vi "DisplayExternals.vi"(7 "AcroPDF":refnum<k7>(container), 8 "error in (no error)":errorcluster, 10 "Dynamic data":T1, 11 "Input parameters":T2={"Measurement type"=enum."Test", "Sensor type"=enum."HPK_8in_256", "Identifier"="test.txt", "Open after execution?"=FALSE, "Plot after execution?"=FALSE, "Display channel"=0, "Voltage Delay (s)"=0.5, "Switch Delay (s)"=0.01, "VISA resource name source"="", "VISA resource name DMM"="", "VISA resource name LCR"="", "Compliance  Level (uA)"=10.0, "Voltage Limit (V)"=1000.0, "Data storage location"="", "Scan voltages"="", "Use source as DMM?"=FALSE, "Single channel?"=FALSE, "LCR signal frequenzy (Hz)"=10.0, "DMM device"=enum."Keithley2001", "Sampling number"=1, "Use env. sensors on"=enum."Sensirion sht1x/7x"} {"Voltage Limit (V)" format="%#_13g"; "Voltage Delay (s)" format="%#_13g"; "Switch Delay (s)" format="%#_13g"}) -> (0 "error out":errorcluster, 2 "Dynamic data":T1, 3 "Input parameters":T2={"Measurement type"=enum."Test", "Sensor type"=enum."HPK_8in_256", "Identifier"="test.txt", "Open after execution?"=FALSE, "Plot after execution?"=FALSE, "Display channel"=0, "Voltage Delay (s)"=0.5, "Switch Delay (s)"=0.01, "VISA resource name source"="", "VISA resource name DMM"="", "VISA resource name LCR"="", "Compliance  Level (uA)"=10.0, "Voltage Limit (V)"=1000.0, "Data storage location"="", "Scan voltages"="", "Use source as DMM?"=FALSE, "Single channel?"=FALSE, "LCR signal frequenzy (Hz)"=10.0, "DMM device"=enum."Keithley2001", "Sampling number"=1, "Use env. sensors on"=enum."Sensirion sht1x/7x"} {"Voltage Limit (V)" format="%#_13g"; "Voltage Delay (s)" format="%#_13g"; "Switch Delay (s)" format="%#_13g"})   [LabVIEW 2016]
uses:
  Input_parameters.ctl
  Dynamic_data.ctl
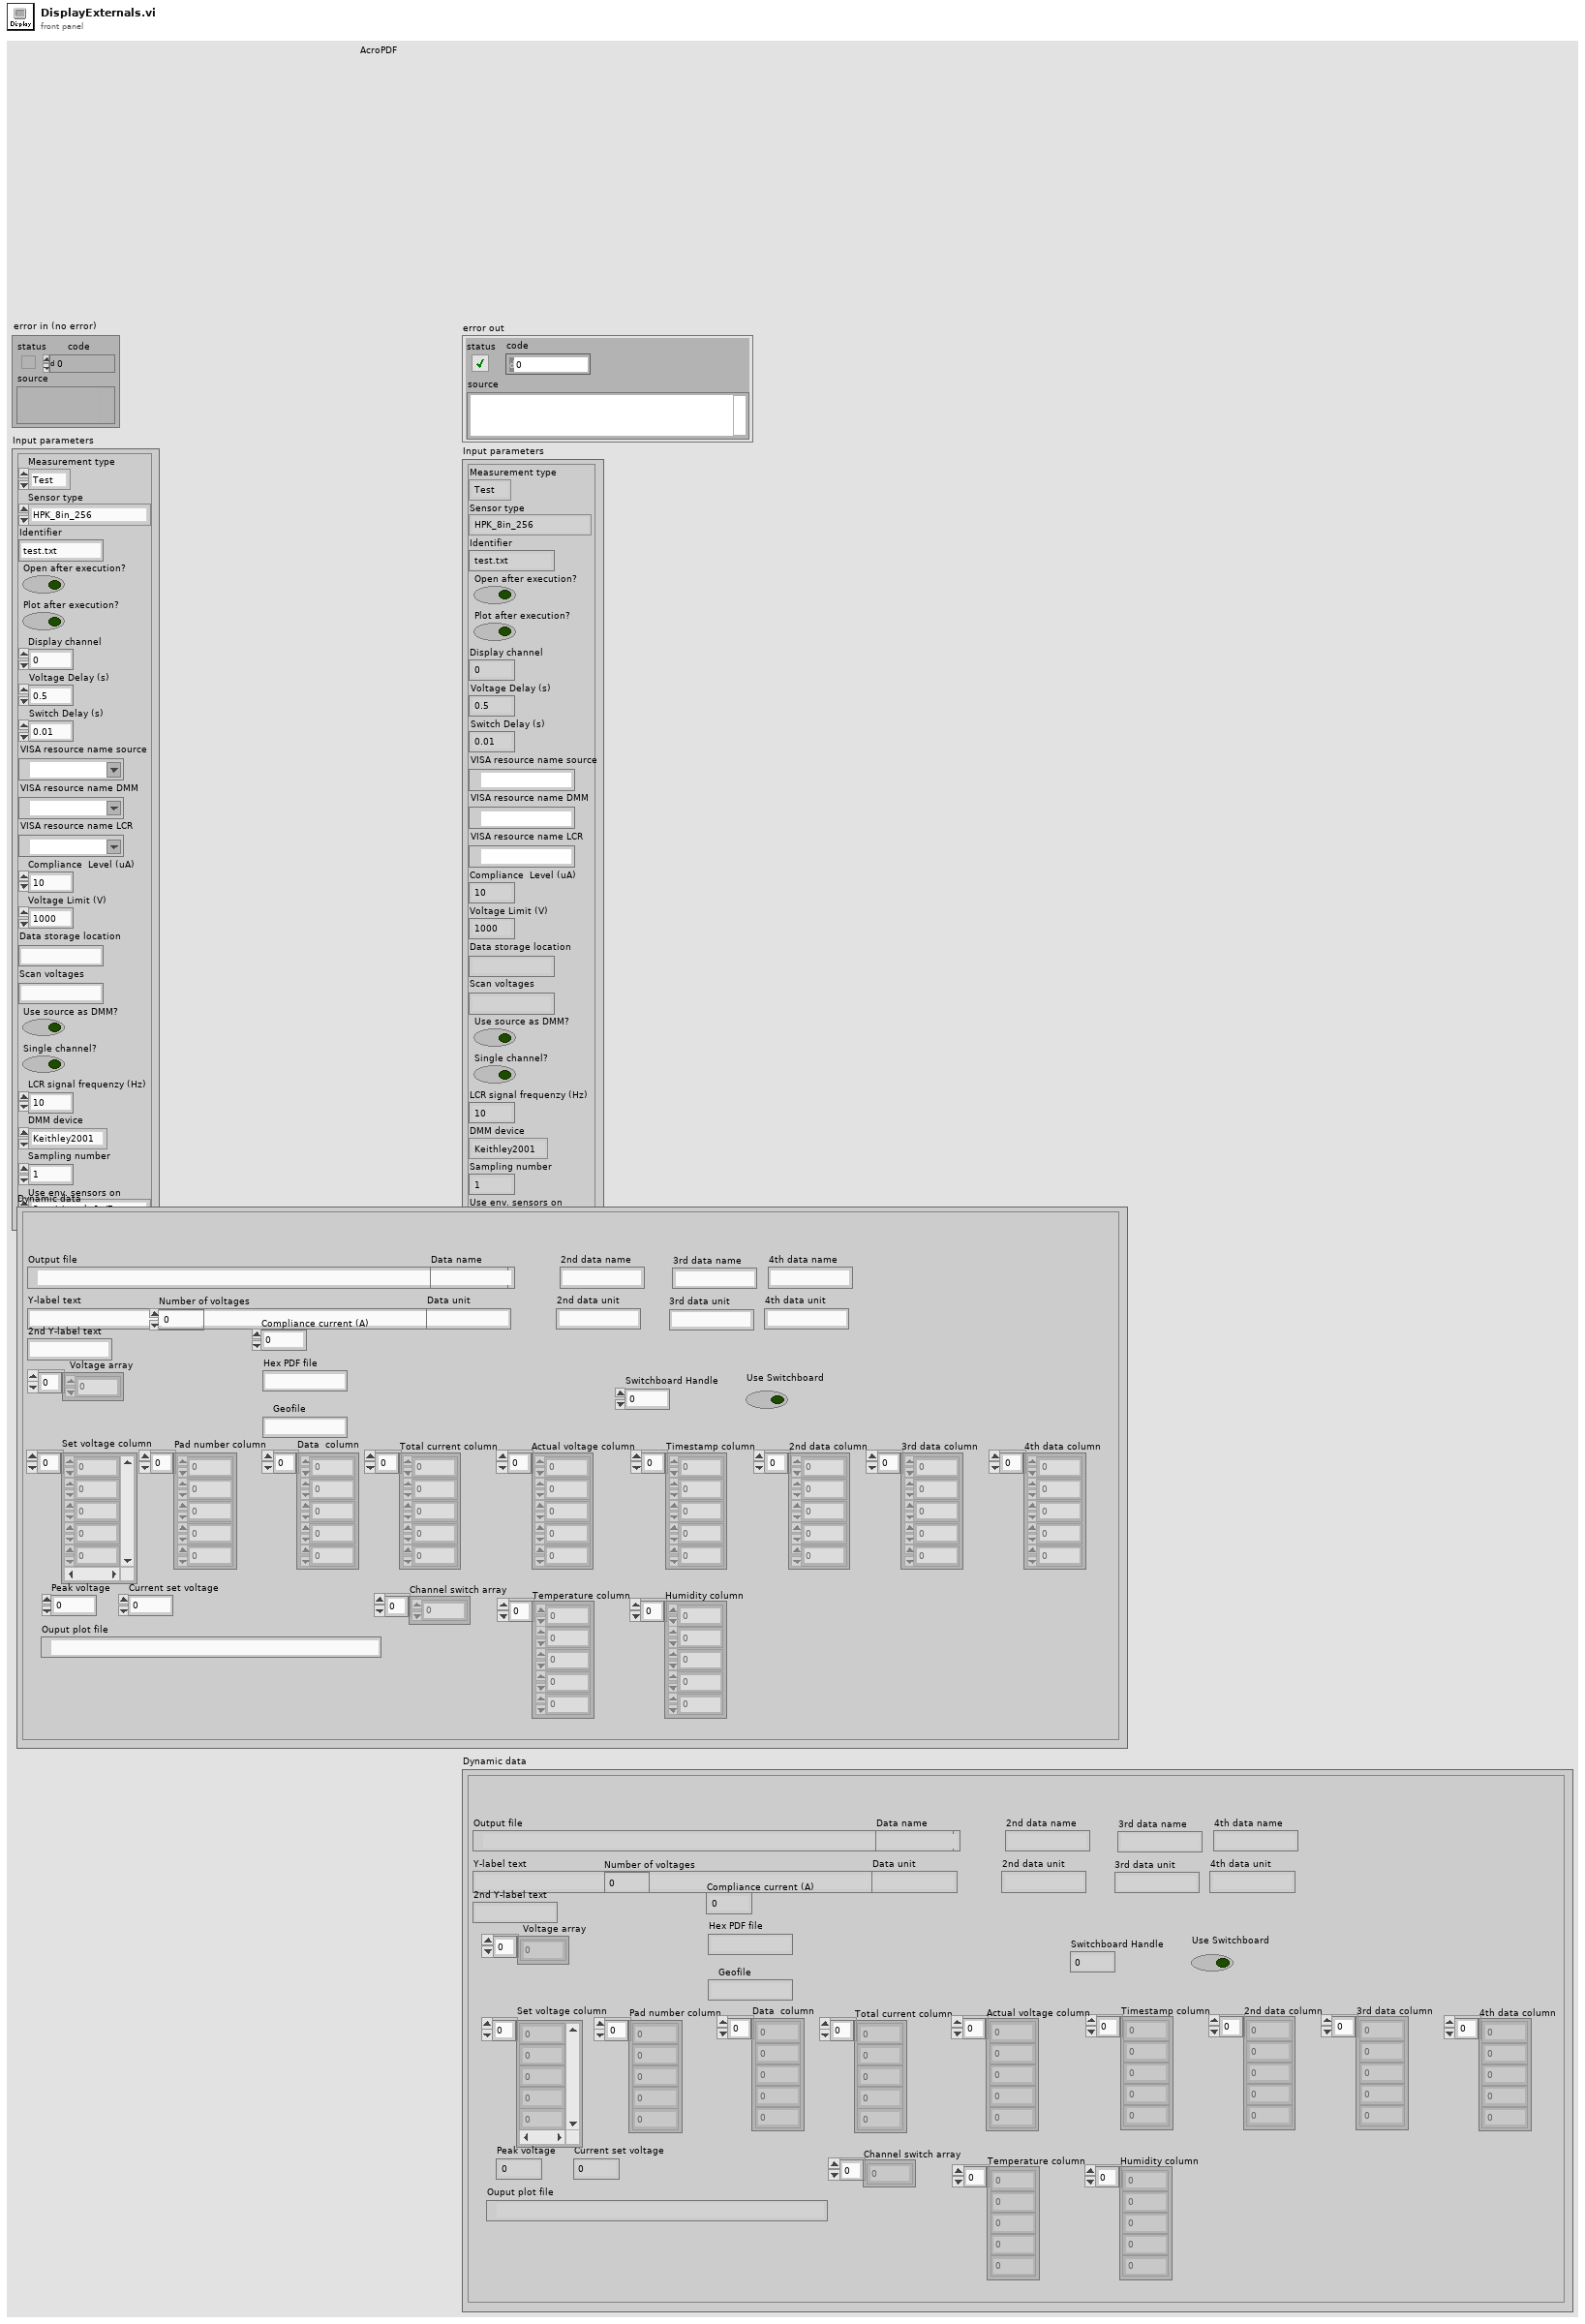
[diagram p1: front panel]
types:
  T1 = typedef "Dynamic_data.ctl" = cluster{"Output file":path, "Y-label text":string, "Current set voltage":dbl, "Set voltage column":dbl[], "Pad number column":dbl[], "Data  column":dbl[], "Number of voltages":i32, "Compliance current (A)":dbl, "Geofile":string, "Peak voltage":dbl, "Hex PDF file":string, "Voltage array":dbl[], "Total current column":dbl[], "Timestamp column":dbl[], "Data name":string, "Data unit":string, "2nd data column":dbl[], "2nd data name":string, "2nd data unit":string, "3rd data column":dbl[], "4th data column":dbl[], "3rd data name":string, "3rd data unit":string, "4th data name":string, "4th data unit":string, "Actual voltage column":dbl[], "2nd Y-label text":string, "Ouput plot file":path, "Temperature column":dbl[], "Humidity column":dbl[], "Switchboard Handle":u32, "Use Switchboard":bool, "Channel switch array":i32[]}
  T2 = typedef "Input_parameters.ctl" = cluster{"Measurement type":enum16{"IV", "CV", "Test"}, "Sensor type":enum16{"HPK_6in_135", "HPK_8in_256", "INF_8in_256", "Diode", "HPK_6in_256", "Test capacitances"}, "Identifier":string, "Open after execution?":bool, "Plot after execution?":bool, "Display channel":i32, "Voltage Delay (s)":dbl, "Switch Delay (s)":dbl, "VISA resource name source":refnum<visa-resource-name>, "VISA resource name DMM":refnum<visa-resource-name>, "VISA resource name LCR":refnum<visa-resource-name>, "Compliance  Level (uA)":dbl, "Voltage Limit (V)":dbl, "Data storage location":string, "Scan voltages":string, "Use source as DMM?":bool, "Single channel?":bool, "LCR signal frequenzy (Hz)":dbl, "DMM device":enum16{"Keithley2001", "Keithley2450", "Keithley2410", "Keithley6487"}, "Sampling number":i32, "Use env. sensors on":enum16{"Sensirion sht1x/7x", "Switch Matrix", "Probecard"}}
  T3 = enum16{"HPK_6in_135", "HPK_8in_256", "INF_8in_256", "Diode", "HPK_6in_256", "Test capacitances"}
  T4 = typedef "imagedata.ctl" = cluster{"image type":i32, "image depth":i32, "image":u8[], "mask":u8[], "colors":u32[], "Rectangle":cluster{"left":i16, "top":i16, "right":i16, "bottom":i16}}
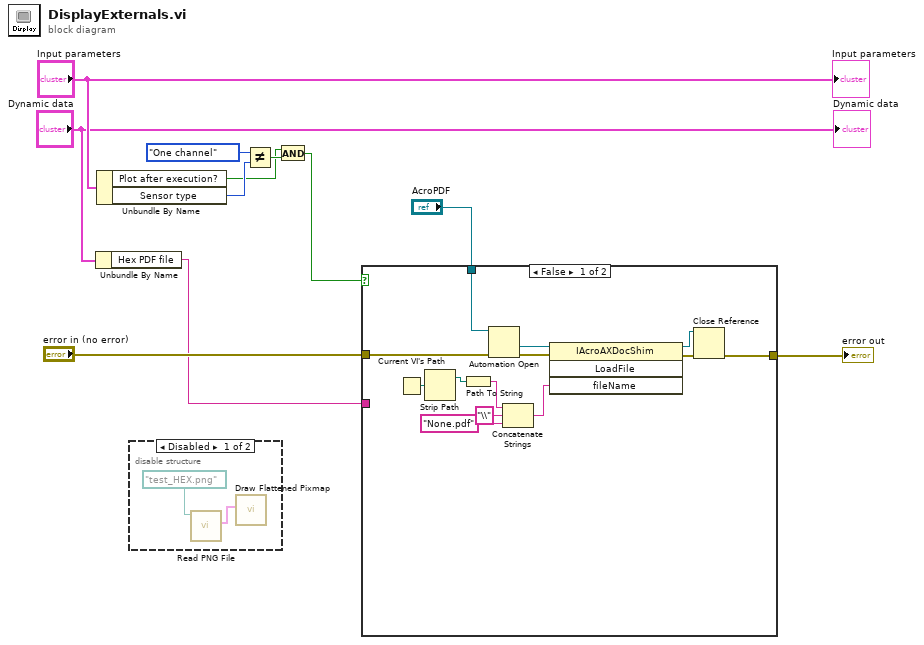
[diagram p0: block diagram]
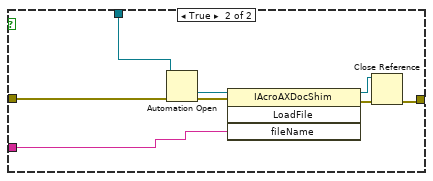
[diagram p3: hidden frame]
diagram:
  n1 = Unbundle By Name("Dynamic data") -> ("Hex PDF file"=w7:string)
  n2 = Unbundle By Name("Input parameters") -> ("Plot after execution?"=w3:bool, "Sensor type"=w6:T3)
  n3 = disable-structure shown="Disabled" {
    frame Disabled {
      n4 = call <vilib>:"Read PNG File.vi"("path to PNG file"=path "test_HEX.png") -> ("image data"=w14:T4)  [unwired: 8 in, 2 out]
      n5 = call <vilib>:"Draw Flattened Pixmap.vi"("image data"=w14) -> ("new picture"=w12:picture)  [unwired: 8 in]
    }
    frame Enabled {
    }
  }
  n6 = Not Equal?(x=enum16{"6''", "8''", "One channel"}."One channel", y=w6) -> (x != y?=w4:bool)
  n7 = And(x=w3, y=w4) -> (x .and. y?=w2:bool)
  n8 = case shown="False" w2 {
    tunnel: "error in (no error)" -> [w16 w29]
    tunnel: [w23 w35] -> w10
    tunnel: "AcroPDF" -> [w15 w34]
    tunnel: w7 -> [_ w28]
    frame False {
      n9 = Current VI's Path() -> (path=w20:path)
      n10 = Strip Path(path=w20) -> (stripped path=w19:path)  [unwired: 1 out]
      n11 = Path To String(path=w19) -> (string=w18:string)
      n12 = Automation Open(error in (no error)=w16, Automation Refnum=w15) -> (Automation Refnum=w27:refnum<k7>, error out=w26:errorcluster)  [unwired: 2 in]
      n13 = Concatenate Strings(w18, "\\" ("string"), "None.pdf" ("string")) -> (w17:string)
      n14 = invoke class="IAcroAXDocShim" method="LoadFile"(reference=w27, error in=w26, "fileName"=w17) -> (reference out=w25:refnum<k7>, error out=w24:errorcluster)  [unwired: 1 in, 2 out]
      n15 = Close Reference(reference=w25, error in (no error)=w24) -> (error out=w23:errorcluster)
    }
    frame True {
      n16 = Automation Open(error in (no error)=w29, Automation Refnum=w34) -> (Automation Refnum=w33:refnum<k7>, error out=w32:errorcluster)  [unwired: 2 in]
      n17 = invoke class="IAcroAXDocShim" method="LoadFile"(reference=w33, error in=w32, "fileName"=w28) -> (reference out=w31:refnum<k7>, error out=w30:errorcluster)  [unwired: 1 in, 2 out]
      n18 = Close Reference(reference=w31, error in (no error)=w30) -> (error out=w35:errorcluster)
    }
  }
  "error out" <- w10
  "Input parameters" <- "Input parameters"
  "Dynamic data" <- "Dynamic data"
